vi "Match equation target to real life.vi"(2 "Camera angle":dbl, 3 "Height from camera":dbl, 4 "Calculated height":dbl) -> (0 "Distance from Camera":dbl, 1 "Angle on Camera":dbl)   [LabVIEW 2012]
panel:
  # "The watched angle for the same point"
  # "To center of the target"
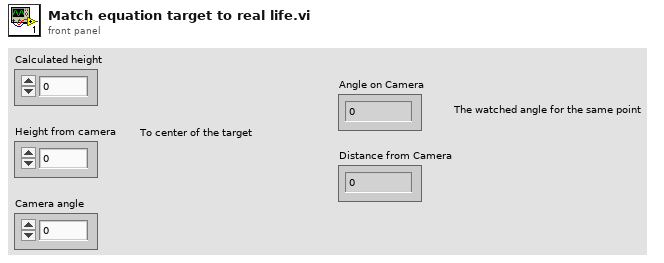
[diagram p1: front panel]
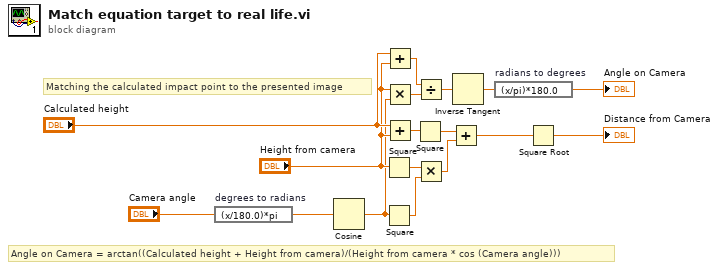
[diagram p0: block diagram]
diagram:
  # "Matching the calculated impact point to the presented image"
  # "Angle on Camera = arctan((Calculated height + Height from camera)/(Height from camera * cos (Camera angle)))"
  n1 = expression code="(x/180.0)*pi" "degrees to radians"("Camera angle") -> (w13:dbl)
  n2 = Cosine(x=w13) -> (cos(x)=w6:dbl)
  n3 = Square(x="Height from camera") -> (x^2=w5:dbl)
  n4 = Square(x=w6) -> (x^2=w4:dbl)
  n5 = Add(x="Calculated height", y="Height from camera") -> (x+y=w15:dbl)
  n6 = Multiply(x="Height from camera", y=w6) -> (x*y=w12:dbl)
  n7 = Add(x="Calculated height", y="Height from camera") -> (x+y=w8:dbl)
  n8 = Square(x=w8) -> (x^2=w3:dbl)
  n9 = Divide(x=w15, y=w12) -> (x/y=w11:dbl)
  n10 = Multiply(x=w5, y=w4) -> (x*y=w2:dbl)
  n11 = Add(x=w3, y=w2) -> (x+y=w1:dbl)
  n12 = Inverse Tangent(1:w11) -> (0:w16:dbl)
  n13 = expression code="(x/pi)*180.0" "radians to degrees"(w16) -> (→"Angle on Camera":dbl)
  n14 = Square Root(x=w1) -> (sqrt(x)=→"Distance from Camera":dbl)
